vi "getfreqandpwr.vi"(11 "Comm Handle":u32) -> (0 "Freq":dbl format="%.7f", 3 "RF Detector Pwr dBm":dbl=-67.9609375 format="%_5g", 4 "error?":bool, 8 "EOS":bool)   [LabVIEW 2013]
uses:
  <vilib>/Utility/error.llb/DialogType.ctl
  instr.lib/lvserial/lvserial.lvlib
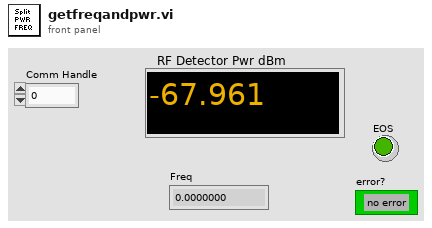
[diagram p1: front panel]
types:
  T1 = typedef "DialogType.ctl" = u16
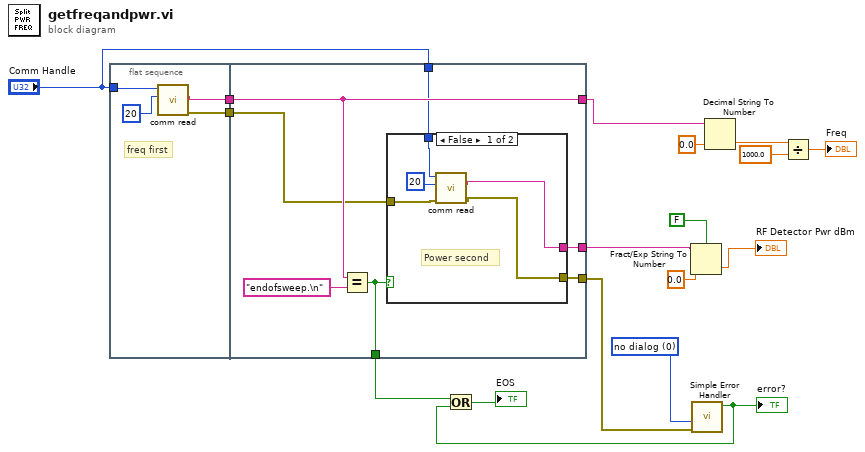
[diagram p0: block diagram]
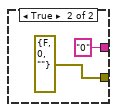
[diagram p2: hidden frame]
diagram:
  w6 = T1 0 items=["no dialog", "OK message", "continue or stop message", "OK message + warnings", "continue/stop + warnings"] ("type of dialog (OK msg:1)")
  n1 = flat-sequence {
    tunnel: "Comm Handle" -> [w21]
    tunnel: [w18] -> w13
    tunnel: [w19] -> w8
    tunnel: [w25] -> w12
    tunnel: w13 -> [w25]
    tunnel: [w27] -> w5
    tunnel: [w26] -> w11
    tunnel: "Comm Handle" -> [w24]
    tunnel: w8 -> [w23]
    tunnel: [w22] -> w7
    frame #0 {
      # "freq first"
      n2 = call "comm read.vi"("requested byte count"=u32 20 ("byte count"), "Comm Handle"=w21) -> ("error out"=w19:errorcluster, "string read"=w18:string)  [unwired: 6 in, 2 out]
    }
    frame #1 {
      n3 = Equal?(x=w25, y="endofsweep.\n") -> (x = y?=w27:bool)
      n4 = case shown="False" w27 {
        tunnel: [w30 "0" ("read buffer")] -> w26
        tunnel: w24 -> [w33 _]
        tunnel: w23 -> [w31 _]
        tunnel: [w29 errorcluster {"status"=FALSE, "code"=0, "source"=""} ("error out")] -> w22
        frame False {
          # "Power second"
          n5 = call "comm read.vi"("error in (no error)"=w31, "requested byte count"=u32 20 ("byte count"), "Comm Handle"=w33) -> ("error out"=w29:errorcluster, "string read"=w30:string)  [unwired: 5 in, 2 out]
        }
        frame True {
        }
      }
    }
  }
  n6 = Fract/Exp String To Number(use system decimal point (T)=FALSE, string=w11, default (0 dbl)=0.0 ("default (0 I32)")) -> (number=→"RF Detector Pwr dBm":dbl)  [unwired: 1 in, 1 out]
  n7 = call <vilib>:"Simple Error Handler.vi"("type of dialog (OK msg:1)"=w6, "error in (no error)"=w7) -> ("error?"=w3:bool)  [unwired: 7 out]
  "error?" <- w3
  n8 = Or(x=w5, y=w3) -> (x .or. y?=→"EOS":bool)
  n9 = Decimal String To Number(string=w12, default (0L)=0.0 ("default (0 I32)")) -> (number=w17:dbl)  [unwired: 1 in, 1 out]
  n10 = Divide(x=w17, y=1000.0) -> (x/y=→"Freq":dbl)
